vi "PPL_ActionVIOnRecompile_InlineAsync.vi"(8 "error in":errorcluster, 9 "Timeout (ms)":u32, 10 "Runtime Configurable Section Path":string, 11 "Device Item Ref in":T1 format="%.0x") -> (0 "error out":errorcluster)   [LabVIEW 2020]
uses:
  <vilib>/NI VeriStand/Custom Device API/Custom Device Item Ref.ctl
  <vilib>/NI VeriStand/Custom Device API/Custom Device Channel Type.ctl
  <vilib>/NI VeriStand/Custom Device API/Block Data Reference.ctl
  <vilib>/NI VeriStand/Custom Device API/Data Reference.ctl
  <vilib>/NI VeriStand/Custom Device API/Get Item Property (U16).vi
  <vilib>/NI VeriStand/Custom Device API/Get Item Property (Variant).vi
  <vilib>/NI VeriStand/Execution/CustomDevice/NI VeriStand - Send Custom Device Message (Byte Array).vi
  <vilib>/NI VeriStand/Custom Device API/Custom Device API.lvlib
  <vilib>/NI/NIVS Inline Async API/_Data Access System Explorer/Data Access System Explorer.lvlib
  <vilib>/NI VeriStand/Execution/CustomDevice/NI_VS Custom Device ExecutionAPI.lvlib
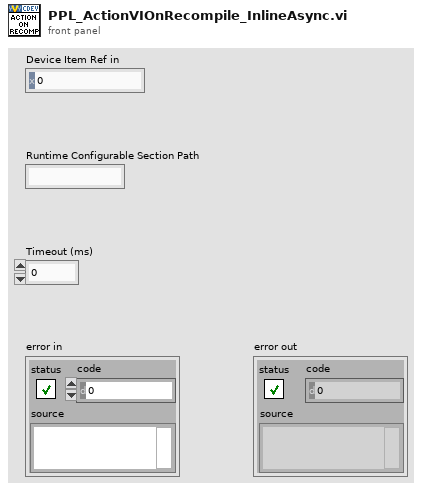
[diagram p1: front panel]
types:
  T1 = typedef "Custom Device API.lvlib/Custom Device Item Ref.ctl" = u64
  T2 = typedef "Custom Device API.lvlib/Custom Device Channel Type.ctl" = enum16{"Input", "Output"}
  T3 = cluster{"Name":string, "Type":enum16{"Output/Write", "Input/Read", "Input/ReadWrite"}, "VS Refs":T1[]}
  T4 = enum16{"Output/Write", "Input/Read", "Input/ReadWrite"}
  T5 = typedef "Custom Device API.lvlib/Block Data Reference.ctl" = cluster{"Data Reference":T6, "Offset":u64, "Length":u64}
  T6 = typedef "Custom Device API.lvlib/Data Reference.ctl" = i32
  T7 = cluster{"Name":string, "Async Init Timeout":u16, "Compiled.InlineAsync.Settings":cluster{"Read":cluster{"Refs":T5[], "Values":dbl[]}[], "Write":cluster{"Refs":T5[], "Values":dbl[]}[], "ReadWrite":cluster{"Refs":T6[], "Values":dbl[], "Reset Values":dbl[]}[], "LUT":variant}}
  T8 = cluster{"Read":cluster{"Refs":T5[], "Values":dbl[]}[], "Write":cluster{"Refs":T5[], "Values":dbl[]}[], "ReadWrite":cluster{"Refs":T6[], "Values":dbl[], "Reset Values":dbl[]}[], "LUT":variant}
  T9 = typedef "Custom Device API.lvlib/Custom Device Item Info.ctl" = cluster{"Name":string, "Is Channel":bool, "GUID":string, "Is Waveform":bool}
  T10 = cluster{"Name":string, "Type":enum16{"Output/Write", "Input/Read", "Input/ReadWrite"}, "VS Refs":T1[]}[]
  T11 = typedef "NI_VS Custom Device ExecutionAPI.lvlib/Custom Device Ref.ctl" = refnum<k24>
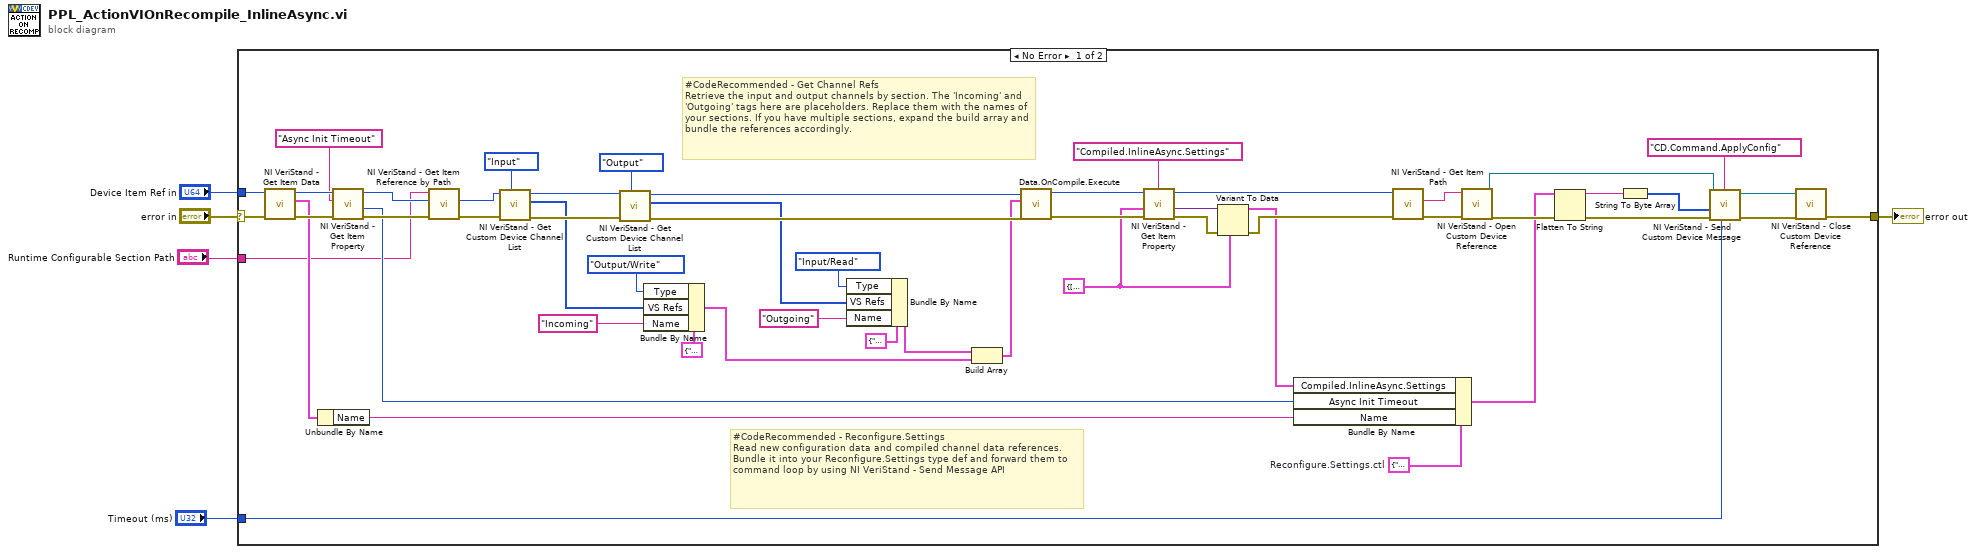
[diagram p0: block diagram]
diagram:
  n1 = case shown="No Error" "error in" {
    selector: "error in" -> [w58 w59]
    tunnel: [w47 w59] -> w4
    tunnel: "Device Item Ref in" -> [w44 _]
    tunnel: "Runtime Configurable Section Path" -> [w28 _]
    tunnel: "Timeout (ms)" -> [w9 _]
    frame No Error {
      w7 = T7 {"Name"="", "Async Init Timeout"=0, "Compiled.InlineAsync.Settings"={"Read"=[], "Write"=[], "ReadWrite"=[], "LUT"=variant}}  # Reconfigure.Settings.ctl
      w15 = T8 {"Read"=[], "Write"=[], "ReadWrite"=[], "LUT"=variant} ("cluster")
      # "#CodeRecommended - Get Channel Refs\nRetrieve the input and output channels by section. The 'Incoming' and 'Outgoing' tags here are placeholders. Replace them with the names of your sections. If you have multiple sections, expand the build array and bundle the references accordingly."
      # "#CodeRecommended - Reconfigure.Settings\nRead new configuration data and compiled channel data references. Bundle it into your Reconfigure.Settings type def and forward them to command loop by using NI VeriStand - Send Message API"
      n2 = call <vilib>:"NI VeriStand - Get Item Data.vi"("error in (no error)"=w58, "Item Ref in"=w44) -> ("error out"=w57:errorcluster, "Item Info"=w43:T9, "Item Ref out"=w32:T1)  [unwired: 6 in, 1 out]
      n3 = Unbundle By Name(w43) -> ("Name"=w42:string)
      n4 = call-poly <vilib>:"NI VeriStand - Get Item Property.vi"("error in (no error)"=w57, "Property Name"="Async Init Timeout", "Item Ref in"=w32) -> ("error out"=w56:errorcluster, "Value"=w30:u16, "Item Ref out"=w29:T1)  [unwired: 5 in, 1 out]
      n5 = call <vilib>:"NI VeriStand - Get Item Reference by Path.vi"("error in (no error)"=w56, "Root Ref"=w29, "Item Path in"=w28) -> ("error out"=w55:errorcluster, "Item Ref"=w27:T1)  [unwired: 5 in, 2 out]
      n6 = call <vilib>:"NI VeriStand - Get Custom Device Channel List.vi"("Channel Type"=Custom_Device_Channel_Type."Input", "error in (no error)"=w55, "Device Ref in"=w27) -> ("error out"=w54:errorcluster, "Specified Channel Ref List"=w23:T1[], "Device Ref out"=w24:T1)  [unwired: 6 in]
      n7 = call <vilib>:"NI VeriStand - Get Custom Device Channel List.vi"("Channel Type"=Custom_Device_Channel_Type."Output", "error in (no error)"=w54, "Device Ref in"=w24) -> ("error out"=w53:errorcluster, "Specified Channel Ref List"=w22:T1[], "Device Ref out"=w21:T1)  [unwired: 6 in]
      n8 = Bundle By Name(cluster=T3 {"Name"="", "Type"=enum."Output/Write", "VS Refs"=[]} ("Group"), "Type"=T4."Output/Write", "VS Refs"=w23, "Name"="Incoming" ("Item Name")) -> (w33:T3)
      n9 = Bundle By Name(cluster=T3 {"Name"="", "Type"=enum."Output/Write", "VS Refs"=[]} ("Group"), "Type"=T4."Input/Read", "VS Refs"=w22, "Name"="Outgoing" ("Item Name")) -> (w38:T3)
      n10 = Build Array(w38, w33) -> (w36:T10)
      n11 = call <vilib>:"Data.OnCompile.Execute.vi"("error in"=w53, "VS Ref Groups"=w36, "Custom Device Ref"=w21) -> ("error out"=w50:errorcluster, "Custom Device Ref"=w17:T1)  [unwired: 7 in]
      n12 = call-poly <vilib>:"NI VeriStand - Get Item Property.vi"("error in (no error)"=w50, "Default Value"=w15, "Property Name"="Compiled.InlineAsync.Settings", "Item Ref in"=w17) -> ("error out"=w45:errorcluster, "Value"=w14:variant, "Item Ref out"=w8:T1)  [unwired: 4 in, 1 out]
      n13 = Variant To Data(error in=w45, type=w15, Variant=w14) -> (data=w6:T8, error out=w52:errorcluster)
      n14 = Bundle By Name(cluster=w7, "Compiled.InlineAsync.Settings"=w6, "Async Init Timeout"=w30, "Name"=w42) -> (w13:T7)
      n15 = call <vilib>:"NI VeriStand - Get Item Path.vi"("error in (no error)"=w52, "Item Ref in"=w8) -> ("error out"=w51:errorcluster, "Path"=w20:string)  [unwired: 6 in, 2 out]
      n16 = call <vilib>:"NI VeriStand - Open Custom Device Reference.vi"("error in (no error)"=w51, "Custom Device Path"=w20) -> ("error out"=w49:errorcluster, "Custom Device"=w19:T11)  [unwired: 8 in]
      n17 = Flatten To String(anything=w13, error in (no error)=w49) -> (data string=w12:string, error out=w48:errorcluster)  [unwired: 2 in, 1 out]
      n18 = String To Byte Array(string=w12) -> (unsigned byte array=w11:u8[])
      n19 = call-poly <vilib>:"NI VeriStand - Send Custom Device Message.vi"("Timeout ms (5000)"=w9, "error in (no error)"=w48, "Data"=w11, "Command"="CD.Command.ApplyConfig", "Custom Device in"=w19) -> ("error out"=w46:errorcluster, "Custom Device out"=w10:T11)  [unwired: 4 in, 1 out]
      n20 = call <vilib>:"NI VeriStand - Close Custom Device Reference.vi"("error in (no error)"=w46, "Custom Device"=w10) -> ("error out"=w47:errorcluster)  [unwired: 9 in]
    }
    frame Error {
    }
  }
  "error out" <- w4
